vi "Main.vi"() -> ()   [LabVIEW 2020]
uses:
  <instrlib>/CAEN PSM/CAEN PSM.lvlib
panel:
  in  "User":string
  out "Ch1 Leak Current":dbl
  out "Ch0 Leak Current":dbl
  in  "Time Between \nTests (minutes)":dbl
  out "Voltage Ch 1":dbl
  out "Voltage Ch 0":dbl
  out "Current Ch 1":dbl
  out "Current Ch 0":dbl
  out "Engaged Tube Ch 1":string
  out "Engaged Tube Ch 0":string
  out "Performing Trip Tests":bool
  out "Current High":bool
  out "Ch 1":dbl[](array[numeric])
  out "Ch 0":dbl[](array[numeric])
  out "POWER TRIPPED":bool
  out "Number of Tests Taken":i32
  out "Array Bad Tubes 2":bool[](array[boolean])
  out "Array Bad Tubes 1":bool[](array[boolean])
  in  "Stop":bool
  in  "Power Supply \nAddress":refnum<visa-resource-name>="ASRL6::INSTR"
  in  "Barcodes in 2":string[](array[string])
  in  "Barcodes in":string[](array[string])
  out "Test Is Running (Red)\nTest Is Stopped (Green)":bool
  in  "Start":bool
  # "*Start with switch flipped\n  to \"Stop Next Iteration\" \n  if you want 1 iteration."
  # "Stop Next\nIteration"
  # "Dark Current Test"
  # "- Load 8 or 16 tubes\n\n- Fill tubes with gas\n\n- Ensure 24V power supply is on\n\n- Scan in barcodes\n\n- Specify time between tests \n     (typically 5-15min)\n\n- Press start\n\n- Toggle switch to end test after  next iteration\n\n- Bad tubes will be indicated with red LEDs"
  # "Continue"
  # "9"
  # "1"
  # "9"
  # "1"
  # "10"
  # "2"
  # "10"
  # "2"
  # "11"
  # "11"
  # "3"
  # "3"
  # "12"
  # "4"
  # "12"
  # "4"
  # "13"
  # "5"
  # "5"
  # "13"
  # "14"
  # "6"
  # "14"
  # "6"
  # "15"
  # "7"
  # "7"
  # "15"
  # "16"
  # "8"
  # "8"
  # "16"
  # "Greyed out LEDs - Cleared and being tested\nRed LEDs - BAD TUBES\nGreen LEDS - Good Tubes"
  # "Red when power trips\nWhite when no power trip"
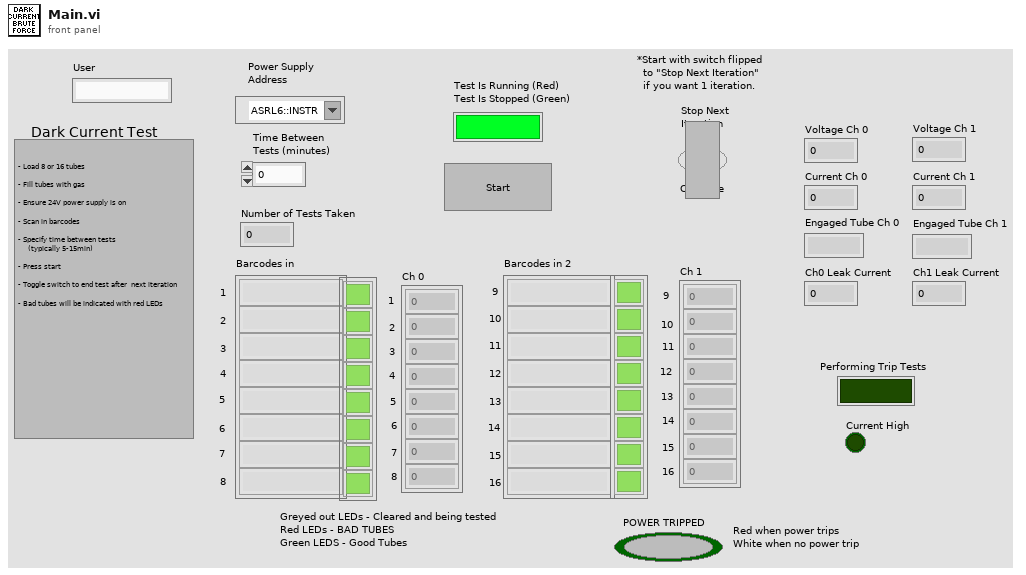
[diagram p1: front panel]
types:
  T1 = enum8{"Enabled", "Disabled", "Disabled and Grayed Out"}
  T2 = cluster{"VISA resource name":refnum<visa-resource-name>, "Board address":u8, "NChannels":u8}
  T3 = typedef "CAEN PSM.lvlib/BoardHandle.ctl" = cluster{"VISA resource name":refnum<visa-resource-name>, "Board address":i8, "NChannels":u8}
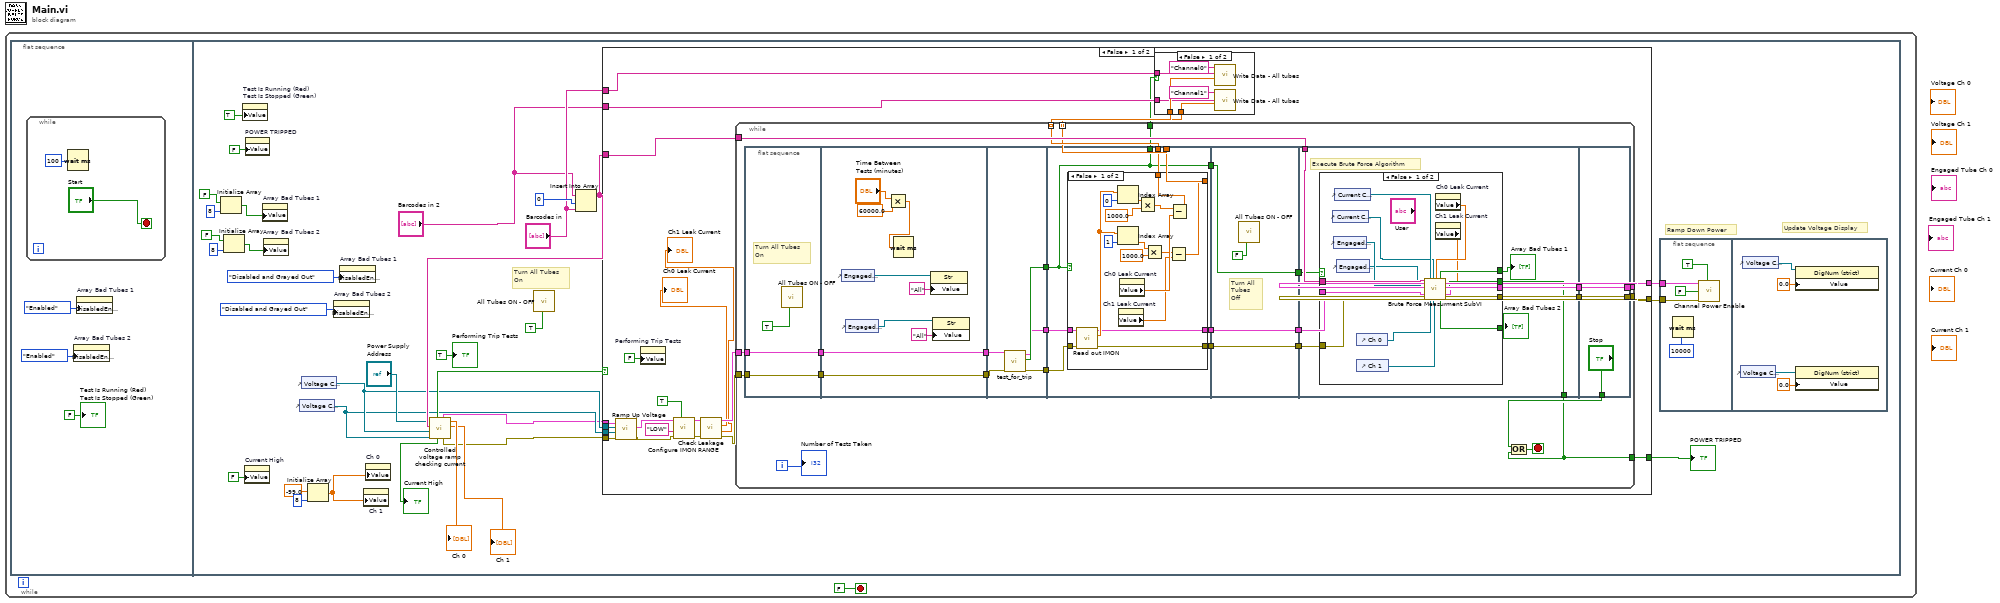
[diagram p0: block diagram]
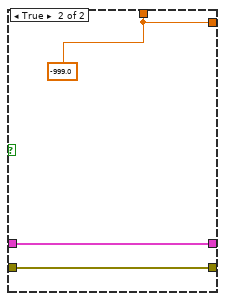
[diagram p3: hidden frame]
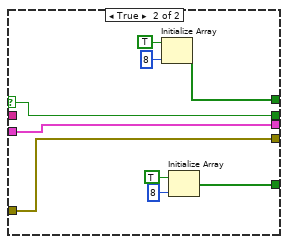
[diagram p4: hidden frame]
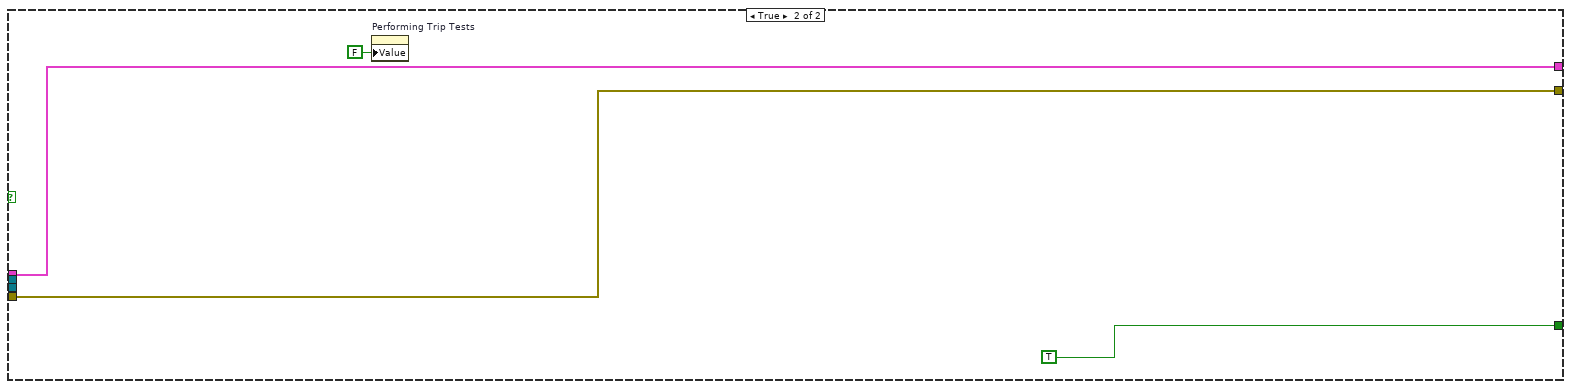
[diagram p5: hidden frame]
diagram:
  n1 = while {
    stop <- FALSE stop-if-true
    n2 = flat-sequence {
      frame #0 {
        n3 = while {
          stop <- "Start" stop-if-true
          n4 = Wait (ms)(milliseconds to wait=u32 100) -> ()  [unwired: 1 out]
        }
        n5 = property on="Array Bad Tubes 2" class="Arr (strict)"("DisabledEnum"=T1."Enabled" ("Disabled")) -> ()  [unwired: 2 in, 2 out]
        n6 = property on="Array Bad Tubes 1" class="Arr (strict)"("DisabledEnum"=T1."Enabled" ("Disabled")) -> ()  [unwired: 2 in, 2 out]
        "Test Is Running (Red)\nTest Is Stopped (Green)" <- FALSE ("Start LED")
      }
      frame #1 {
        # "Update Voltage Display"
        # "Ramp Down Power"
        # "Turn All Tubes \nOn"
        n7 = Initialize Array(FALSE, 8 ("dimension size")) -> (w29:bool[])
        n8 = Initialize Array(FALSE, 8 ("dimension size")) -> (w28:bool[])
        n9 = property on="Test Is Running (Red)\nTest Is Stopped (Green)" class="Bool (strict)"("Value"=TRUE) -> ()  [unwired: 2 in, 2 out]
        n10 = property on="Current High" class="Bool (strict)"("Value"=FALSE ("Current High")) -> ()  [unwired: 2 in, 2 out]
        n11 = property on="POWER TRIPPED" class="Bool (strict)"("Value"=FALSE) -> ()  [unwired: 2 in, 2 out]
        n12 = property on="Array Bad Tubes 1" class="Arr (strict)"("Value"=w29) -> ()  [unwired: 2 in, 2 out]
        n13 = property on="Array Bad Tubes 2" class="Arr (strict)"("Value"=w28) -> ()  [unwired: 2 in, 2 out]
        n14 = control-ref of="Voltage Ch 1"() -> (w12:refnum<vi>)
        n15 = control-ref of="Voltage Ch 0"() -> (w13:refnum<vi>)
        n16 = Initialize Array(-99.0 ("element"), 8 ("dimension size")) -> (w14:dbl[])
        n17 = property on="Array Bad Tubes 2" class="Arr (strict)"("DisabledEnum"=T1."Disabled and Grayed Out" ("Disabled")) -> ()  [unwired: 2 in, 2 out]
        n18 = property on="Array Bad Tubes 1" class="Arr (strict)"("DisabledEnum"=T1."Disabled and Grayed Out" ("Disabled")) -> ()  [unwired: 2 in, 2 out]
        n19 = property on="Ch 1" class="Arr (strict)"("Value"=w14) -> ()  [unwired: 2 in, 2 out]
        n20 = property on="Ch 0" class="Arr (strict)"("Value"=w14) -> ()  [unwired: 2 in, 2 out]
        n21 = call "All Tubes ON - OFF.vi"("Tubes ON/OFF"=TRUE) -> ()  [unwired: 11 in]
        n22 = Insert Into Array(array="Barcodes in 2", index=0, new element="Barcodes in") -> (w24:string[])
        n23 = call "Controlled voltage ramp checking current.vi"("V Ch 1"=w12, "V Ch 0"=w13, "Barcodes in"=w24, "VISA Refnum in"="Power Supply \nAddress") -> ("Ch 2 High"=→"Ch 1":dbl[], "Ch 1 High"=→"Ch 0":dbl[], "error out"=w7:errorcluster, "BoardHandle out 3"=w8:T2, "Current High"=→"Current High":bool, "Power Trip"=w21:bool)  [unwired: 2 out]
        n24 = case shown="False" w21 {
          tunnel: [w62 w183] -> w35
          tunnel: [w61 w184] -> w34
          tunnel: w8 -> [w55 w184]
          tunnel: w7 -> [w56 w183]
          tunnel: w24 -> [w60 _]
          tunnel: w13 -> [w45 _]
          tunnel: w12 -> [w46 _]
          tunnel: "Barcodes in" -> [w50 _]
          tunnel: "Barcodes in 2" -> [w49 _]
          tunnel: [w48 TRUE] -> w10
          frame False {
            n25 = call "Ramp Up Voltage.vi"("error in"=w56, "V Ch 1"=w46, "V Ch 0"=w45, "BoardHandle in"=w55) -> ("error out"=w57:errorcluster, "BoardHandle out"=w54:T2)  [unwired: 6 in]
            n26 = property on="Performing Trip Tests" class="Bool (strict)"("Value"=FALSE ("Performing Trip Tests")) -> ()  [unwired: 2 in, 2 out]
            n27 = call <instrlib>:"Configure IMON RANGE.vi"("All Channels (F)"=TRUE, "error in (no error)"=w57, "IMon range (LOW)"="LOW", "BoardHandle"=w54) -> ("error out"=w41:errorcluster, "BoardHandle out"=w42:T3)  [unwired: 6 in]
            n28 = call "Check Leakage.vi"("error in"=w41, "BoardHandle in"=w42) -> ("error out"=w43:errorcluster, "Ch1 Leak"=→"Ch1 Leak Current":dbl, "Ch0 Leak"=→"Ch0 Leak Current":dbl, "BoardHandle out"=w44:T2)  [unwired: 6 in]
            n29 = while {
              tunnel: w44 -> [w83]
              tunnel: [w94] -> w61
              tunnel: w43 -> [w81]
              tunnel: [w95] -> w62
              tunnel: w60 -> [w93]
              tunnel: [w85] -> w52 mode=indexing
              tunnel: [w84] -> w51 mode=indexing
              tunnel: [w69] -> w48
              tunnel: [w72] -> w47
              i -> [w90]
              stop <- w71 stop-if-true
              n30 = flat-sequence {
                tunnel: w83 -> [w98]
                tunnel: [w98] -> w82
                tunnel: w81 -> [w97]
                tunnel: [w97] -> w80
                tunnel: w82 -> [w103]
                tunnel: w80 -> [w104]
                tunnel: [w104] -> w79
                tunnel: [w103] -> w78
                tunnel: w79 -> [w112]
                tunnel: w78 -> [w111]
                tunnel: [w110] -> w77
                tunnel: [w109] -> w76
                tunnel: [w108] -> w75
                tunnel: [w119] -> w88
                tunnel: [w118] -> w86
                tunnel: [w117] -> w85
                tunnel: [w116] -> w84
                tunnel: w77 -> [w113]
                tunnel: w76 -> [w115]
                tunnel: w75 -> [w114]
                tunnel: [w113] -> w73
                tunnel: [w113] -> w72
                tunnel: [w142] -> w89
                tunnel: w88 -> [w142]
                tunnel: [w141] -> w87
                tunnel: w86 -> [w141]
                tunnel: [w140] -> w74
                tunnel: w73 -> [w140]
                tunnel: w93 -> [w150]
                tunnel: [w152] -> w92
                tunnel: [w151] -> w91
                tunnel: w89 -> [w147]
                tunnel: w87 -> [w146]
                tunnel: w74 -> [w145]
                tunnel: [w144] -> w69
                tunnel: [w179] -> w94
                tunnel: [w180] -> w95
                tunnel: w92 -> [w180]
                tunnel: w91 -> [w179]
                tunnel: ["Stop"] -> w70
                frame #0 {
                  # "Turn All Tubes \nOn"
                  n31 = call "All Tubes ON - OFF.vi"("Tubes ON/OFF"=TRUE) -> ()  [unwired: 11 in]
                }
                frame #1 {
                  n32 = control-ref of="Engaged Tube Ch 0"() -> (w100:refnum<vi>)
                  n33 = control-ref of="Engaged Tube Ch 1"() -> (w99:refnum<vi>)
                  n34 = Multiply(x="Time Between \nTests (minutes)", y=60000.0) -> (x*y=w105:dbl)
                  n35 = Wait (ms)(milliseconds to wait=w105) -> ()  [unwired: 1 out]
                  n36 = property on="Property Node" class="Str"(reference=w100, "Value"="All") -> ()  [unwired: 1 in, 2 out]
                  n37 = property on="Property Node" class="Str"(reference=w99, "Value"="All") -> ()  [unwired: 1 in, 2 out]
                }
                frame #2 {
                  n38 = call "test_for_trip.vi"("error in (no error)"=w112, "BoardHandle in"=w111) -> ("error out"=w108:errorcluster, "Trip?"=w110:bool, "BoardHandle out 3"=w109:T2)  [unwired: 7 in]
                }
                frame #3 {
                  n39 = case shown="False" w113 {
                    tunnel: [w133 w138] -> w119
                    tunnel: [w132 w137] -> w118
                    tunnel: [w124 w139] -> w117
                    tunnel: [w120 w139] -> w116
                    tunnel: w115 -> [w127 w138]
                    tunnel: w114 -> [w126 w137]
                    frame False {
                      n40 = call <instrlib>:"Read out IMON.vi"("error in (no error)"=w126, "BoardHandle"=w127) -> ("error out"=w132:errorcluster, "IMon values (uA)"=w134:dbl[], "BoardHandle out"=w133:T3)  [unwired: 6 in, 1 out]
                      n41 = Index Array(array=w134, index=0) -> (element=w131:dbl)
                      n42 = Index Array(array=w134, index=1) -> (element=w129:dbl)
                      n43 = property on="Ch1 Leak Current" class="DigNum (strict)"() -> ("Value"=w121:dbl)  [unwired: 2 in, 2 out]
                      n44 = property on="Ch0 Leak Current" class="DigNum (strict)"() -> ("Value"=w123:dbl)  [unwired: 2 in, 2 out]
                      n45 = Multiply(x=w131, y=1000.0) -> (x*y=w125:dbl)
                      n46 = Multiply(x=w129, y=1000.0) -> (x*y=w122:dbl)
                      n47 = Subtract(x=w122, y=w121) -> (x-y=w120:dbl)
                      n48 = Subtract(x=w125, y=w123) -> (x-y=w124:dbl)
                    }
                    frame True {
                      w139 = -999.0
                    }
                  }
                }
                frame #4 {
                  # "Turn All \nTubes\nOff"
                  n49 = call "All Tubes ON - OFF.vi"("Tubes ON/OFF"=FALSE ("Activate: 1\nDeactivate: 0")) -> ()  [unwired: 11 in]
                }
                frame #5 {
                  # "Execute Brute Force Algorithm"
                  n50 = case shown="False" w145 {
                    selector: w145 -> [_ w169]
                    tunnel: [w164 w170] -> w152
                    tunnel: [w163 w177] -> w151
                    tunnel: w150 -> [w166 _]
                    tunnel: w147 -> [w165 w177]
                    tunnel: [w168 w176] -> w149
                    tunnel: [w167 w174] -> w148
                    tunnel: w146 -> [w162 w170]
                    tunnel: [w159 w169] -> w144
                    frame False {
                      n51 = control-ref of="Current Ch 1"() -> (w157:refnum<vi>)
                      n52 = control-ref of="Engaged Tube Ch 0"() -> (w156:refnum<vi>)
                      n53 = control-ref of="Current Ch 0"() -> (w158:refnum<vi>)
                      n54 = control-ref of="Engaged Tube Ch 1"() -> (w155:refnum<vi>)
                      n55 = control-ref of="Ch 0"() -> (w161:refnum<vi>)
                      n56 = control-ref of="Ch 1"() -> (w160:refnum<vi>)
                      n57 = property on="Ch1 Leak Current" class="DigNum (strict)"() -> ("Value"=w153:dbl)  [unwired: 2 in, 2 out]
                      n58 = property on="Ch0 Leak Current" class="DigNum (strict)"() -> ("Value"=w154:dbl)  [unwired: 2 in, 2 out]
                      n59 = call "Brute Force Measurment SubVI.vi"("Barcodes in"=w166, "Engaged Tube Ch0"=w156, "Engaged Tube Ch1"=w155, "BoardHandle in"=w165, "error in (no error)"=w162, "Current Ch 0"=w158, "Ch 0 Currents"=w161, "Current Ch 1"=w157, "Ch 1 Currents"=w160, "Channel 0 Leak"=w154, "Channel 1 Leak"=w153) -> ("Bool Bad 1"=w168:bool[], "Bool Bad 2"=w167:bool[], "Trip?"=w159:bool, "BoardHandle out"=w163:T2, "error out"=w164:errorcluster)  [unwired: 3 in, 1 out]
                    }
                    frame True {
                      n60 = Initialize Array(TRUE ("element"), 8 ("dimension size")) -> (w176:bool[])
                      n61 = Initialize Array(TRUE ("element"), 8 ("dimension size")) -> (w174:bool[])
                    }
                  }
                  "Array Bad Tubes 1" <- w149
                  "Array Bad Tubes 2" <- w148
                }
                frame #6 {
                }
              }
              n62 = Or(x=w70, y=w69) -> (x .or. y?=w71:bool)
              "Number of Tests Taken" <- w90
            }
            n63 = case shown="False" w47 {
              tunnel: w52 -> [w68 _]
              tunnel: w51 -> [w67 _]
              tunnel: w50 -> [w66 _]
              tunnel: w49 -> [w65 _]
              frame False {
                n64 = call "Write Data - All tubes.vi"("Array"=w68, "Barcodes"=w66, "Channel Number"="Channel0") -> ()  [unwired: 9 in]
                n65 = call "Write Data - All tubes.vi"("Array"=w67, "Barcodes"=w65, "Channel Number"="Channel1") -> ()  [unwired: 9 in]
              }
              frame True {
              }
            }
          }
          frame True {
            n66 = property on="Performing Trip Tests" class="Bool (strict)"("Value"=FALSE ("Performing Trip Tests")) -> ()  [unwired: 2 in, 2 out]
          }
        }
        "POWER TRIPPED" <- w10
        n67 = flat-sequence {
          tunnel: w35 -> [w189]
          tunnel: w34 -> [w188]
          frame #0 {
            n68 = Wait (ms)(milliseconds to wait=u32 10000) -> ()  [unwired: 1 out]
            n69 = call <instrlib>:"Channel Power Enable.vi"("All Channels (F)"=TRUE, "error in (no error)"=w189, "Enable (OFF)"=FALSE, "BoardHandle"=w188) -> ()  [unwired: 6 in, 2 out]
          }
          frame #1 {
            n70 = control-ref of="Voltage Ch 1"() -> (w192:refnum<vi>)
            n71 = control-ref of="Voltage Ch 0"() -> (w193:refnum<vi>)
            n72 = property class="DigNum (strict)"(reference=w193, "Value"=0.0) -> ()  [unwired: 1 in, 2 out]
            n73 = property class="DigNum (strict)"(reference=w192, "Value"=0.0) -> ()  [unwired: 1 in, 2 out]
          }
        }
        "Performing Trip Tests" <- TRUE ("Performing Trip Tests")
      }
    }
  }
